vi "AddPageContent.vi"(1 "Graph last":bool=TRUE, 2 "Deckblatt":bool, 4 "TableFont":T1[](array[typedef]), 5 "HeaderTableFont":T1={"Font"="Arial", "Size"=10, "Colour"=0, "Bold"=FALSE, "Italic"=FALSE, "Underline"=FALSE, "Strikethrough"=FALSE, "Font Encoding"=enum."Cp1252, WinANSI"}, 6 "Title Font":T1={"Font"="Arial", "Size"=26, "Colour"=0, "Bold"=TRUE, "Italic"=FALSE, "Underline"=TRUE, "Strikethrough"=FALSE, "Font Encoding"=enum."Cp1252, WinANSI"}, 7 "Column Ratio left":sgl[](array[numeric]), 8 "error in":errorcluster, 9 "Graph Array":T3[](array[typedef]) {"Align (Left)" items=["Center", "Justified", "Justified All", "Left", "Right"]}, 10 "Content":T7={"Titel"="Test mit Graph PDF", "Header Table"=[["Murks:", "4711"], ["HolyShit:", "0815"]], "Table Array"=[], "Bemerkungen"=[{"Bemerkung Text"="super geiles PDF", "Align (Left)"=0, "Add Line Feeds (F:No)"=TRUE, "Font"={"Font"="Arial", "Size"=10, "Colour"=0, "Bold"=FALSE, "Italic"=FALSE, "Underline"=FALSE, "Strikethrough"=FALSE, "Font Encoding"=enum."Cp1252, WinANSI"}}, {"Bemerkung Text"="", "Align (Left)"=0, "Add Line Feeds (F:No)"=FALSE, "Font"={"Font"="Arial", "Size"=10, "Colour"=0, "Bold"=FALSE, "Italic"=FALSE, "Underline"=FALSE, "Strikethrough"=FALSE, "Font Encoding"=enum."Cp1252, WinANSI"}}, {"Bemerkung Text"="Tabelle mit optionalen Ergebnissen", "Align (Left)"=3, "Add Line Feeds (F:No)"=FALSE, "Font"={"Font"="Arial", "Size"=10, "Colour"=0, "Bold"=FALSE, "Italic"=FALSE, "Underline"=FALSE, "Strikethrough"=FALSE, "Font Encoding"=enum."Cp1252, WinANSI"}}, {"Bemerkung Text"="Graph geht ab ... ", "Align (Left)"=0, "Add Line Feeds (F:No)"=FALSE, "Font"={"Font"="Arial", "Size"=10, "Colour"=0, "Bold"=FALSE, "Italic"=FALSE, "Underline"=FALSE, "Strikethrough"=FALSE, "Font Encoding"=enum."Cp1252, WinANSI"}}]} {"Table Array"."Horizontal Align" items=["Center", "Justified", "JustifiedAll", "Left", "Right"]; "Table Array"."TablePictures"."Horizontal Align" items=["Center", "Justified", "JustifiedAll", "Left", "Right"]; "Table Array"."Results"."Position" items=["First", "Last"]; "Table Array"."Results"."Horizontal Align" items=["Center", "Justified", "JustifiedAll", "Left", "Right"]; "Bemerkungen"."Align (Left)" items=["Center", "Justified", "Justified All", "Left", "Right"]}, 11 "Context (Eingang)":refnum<class "Context.lvclass">) -> (0 "error out":errorcluster, 3 "Context (Ausgang)":refnum<class "Context.lvclass">)   [LabVIEW 2020, in "PDF Interface.lvlib"]
doc: "To add Content to a PDF Page that was created by \"InitBeforePage\" or after \"AddAdditionalPage\"."
uses:
  PDF Interface.lvlib
  <vilib>/Simplicity AI/SAI_PDF_API/Classes/Context/Controls/SAI_PDF_Font.ctl
  <vilib>/Simplicity AI/SAI_PDF_API/Classes/Context/Controls/SAI_PDF_Font Encoding.ctl
  PDF Interface Helper/PDFContentType.ctl
  PDF Interface Helper/PDFTableContentType.ctl
  PDF Interface Helper/PDFResults.ctl
  PDF Interface Helper/PDFResultPictures.ctl
  PDF Interface Helper/PDFCommentPosition.ctl
  PDF Interface Helper/PDFPageBreak.ctl
  PDF Interface Helper/PDFTablePictures.ctl
  PDF Interface Helper/PDFBemerkung.ctl
  <vilib>/Simplicity AI/SAI_PDF_API/Classes/Context/Controls/SAI_PDF_Text Align.ctl
  PDF Interface Helper/PDFGraph.ctl
  <vilib>/Simplicity AI/SAI_PDF_API/Classes/Context/Context.lvclass
  PDF Interface Helper/PDF Interface Helper.lvlib
panel:
  # "(Cp1252)"
  # "(Cp1252)"
  # "(Cp1252)"
  # "(Cp1252)"
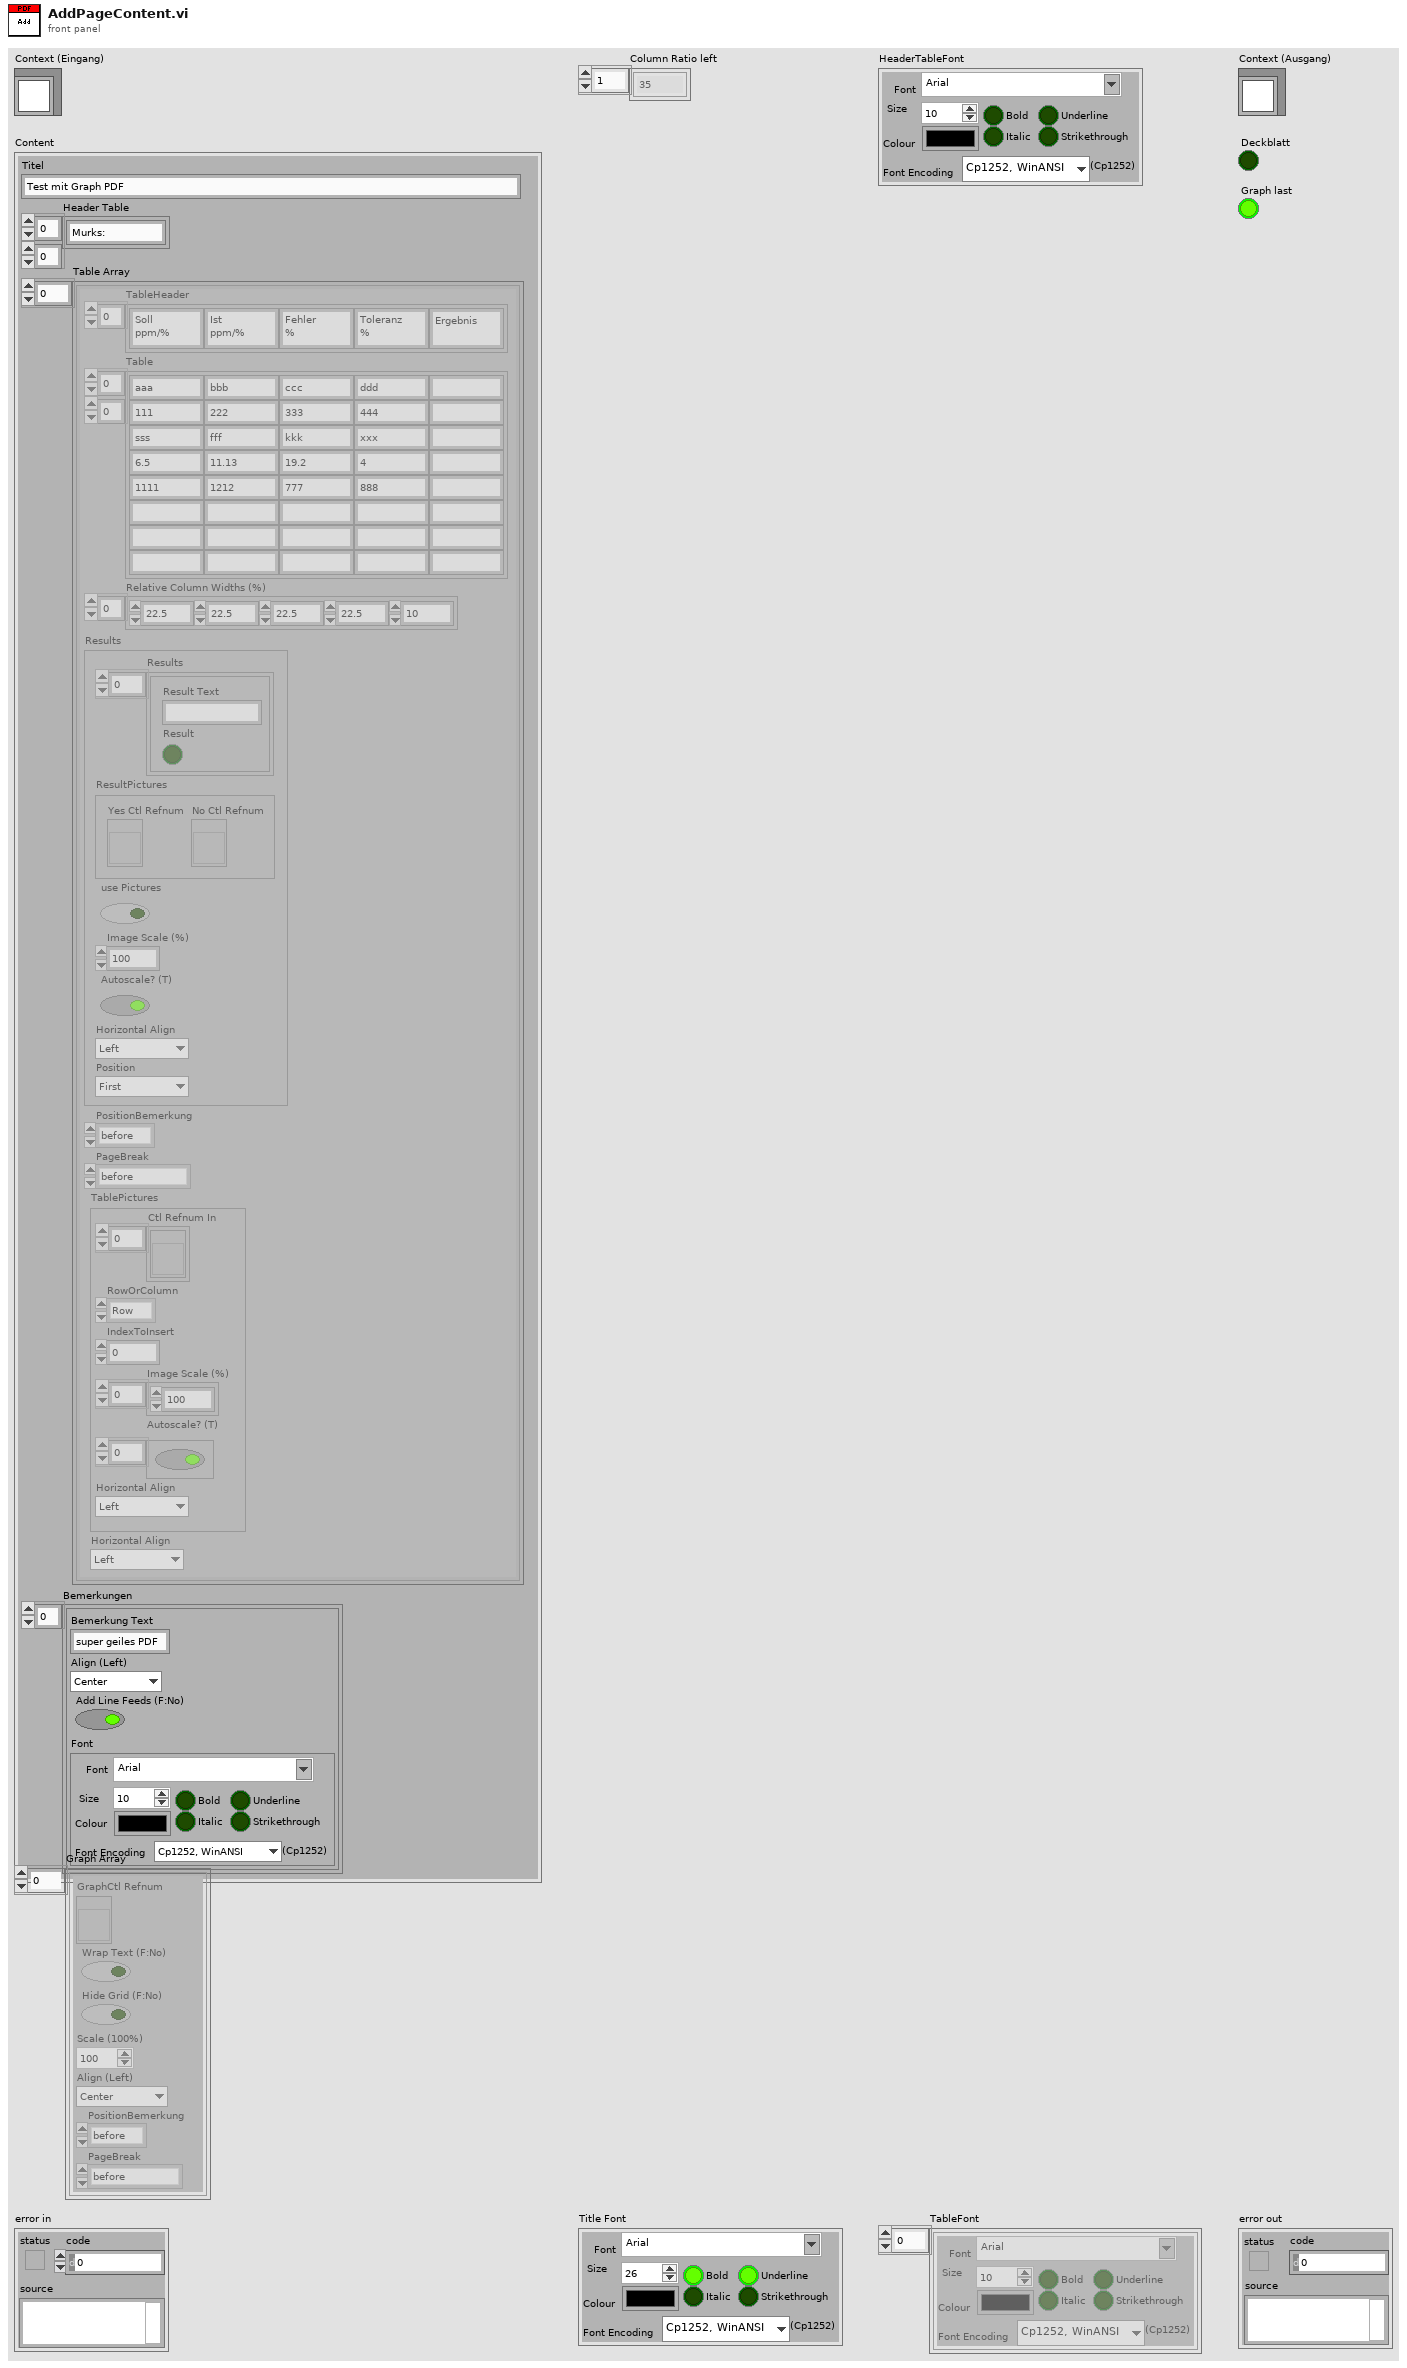
[diagram p1: front panel]
types:
  T1 = typedef "SAI_PDF_Toolkit.lvlib/Context.lvclass/SAI_PDF_Font.ctl" = cluster{"Font":string, "Size":i32, "Colour":u32, "Bold":bool, "Italic":bool, "Underline":bool, "Strikethrough":bool, "Font Encoding":T2}
  T2 = typedef "SAI_PDF_Toolkit.lvlib/Context.lvclass/SAI_PDF_Font Encoding.ctl" = enum16{"Cp1252, WinANSI", "IdentityH", "IdentityV", "Cp1250", "Cp1257", "MacRoman"}
  T3 = typedef "PDF Interface.lvlib/PDF Interface Helper.lvlib/PDFGraph.ctl" = cluster{"GraphCtl Refnum":refnum<vi>, "Wrap Text (F:No)":bool, "Hide Grid (F:No)":bool, "Scale (100%)":sgl, "Align (Left)":T4, "PositionBemerkung":T5, "PageBreak":T6}
  T4 = typedef "SAI_PDF_Toolkit.lvlib/Context.lvclass/SAI_PDF_Text Align.ctl" = i32
  T5 = typedef "PDF Interface.lvlib/PDF Interface Helper.lvlib/PDFCommentPosition.ctl" = enum16{"before", "after"}
  T6 = typedef "PDF Interface.lvlib/PDF Interface Helper.lvlib/PDFPageBreak.ctl" = enum16{"none", "before", "after", "after comment"}
  T7 = typedef "PDF Interface.lvlib/PDF Interface Helper.lvlib/PDFContentType.ctl" = cluster{"Titel":string, "Header Table":string[][], "Table Array":T8[], "Bemerkungen":T12[]}
  T8 = typedef "PDF Interface.lvlib/PDF Interface Helper.lvlib/PDFTableContentType.ctl" = cluster{"TableHeader":string[], "Table":string[][], "Relative Column Widths (%)":sgl[], "Results":T9, "PositionBemerkung":T5, "PageBreak":T6, "TablePictures":T11, "Horizontal Align":i32}
  T9 = typedef "PDF Interface.lvlib/PDF Interface Helper.lvlib/PDFResults.ctl" = cluster{"Results":cluster{"Result Text":string, "Result":bool}[], "ResultPictures":T10, "use Pictures":bool, "Image Scale (%)":sgl, "Autoscale? (T)":bool, "Horizontal Align":i32, "Position":i32}
  T10 = typedef "PDF Interface.lvlib/PDF Interface Helper.lvlib/PDFResultPictures.ctl" = cluster{"Yes Ctl Refnum":refnum<vi>, "No Ctl Refnum":refnum<vi>}
  T11 = typedef "PDF Interface.lvlib/PDF Interface Helper.lvlib/PDFTablePictures.ctl" = cluster{"Ctl Refnum In":refnum<vi>[], "RowOrColumn":enum16{"Row", "Column"}, "IndexToInsert":u16, "Image Scale (%)":sgl[], "Autoscale? (T)":bool[], "Horizontal Align":i32}
  T12 = typedef "PDF Interface.lvlib/PDF Interface Helper.lvlib/PDFBemerkung.ctl" = cluster{"Bemerkung Text":string, "Align (Left)":T4, "Add Line Feeds (F:No)":bool, "Font":T1}
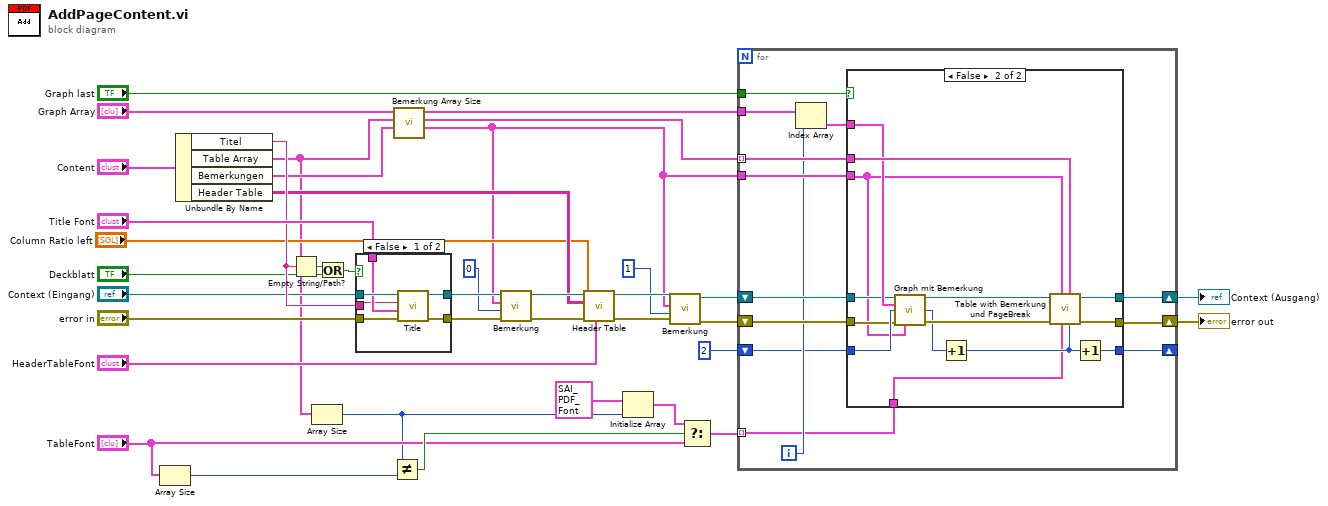
[diagram p0: block diagram]
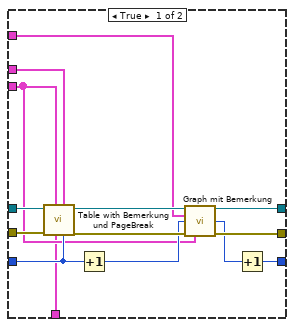
[diagram p2: hidden frame]
diagram:
  n1 = Array Size(array="TableFont") -> (size(s)=w6:i32)
  n2 = Unbundle By Name("Content") -> ("Titel"=w23:string, "Table Array"=w8:T8[], "Bemerkungen"=w12:T12[], "Header Table"=w21:string[][])
  n3 = Empty String/Path?(string/path=w23) -> (empty?=w22:bool)
  n4 = Array Size(array=w8) -> (size(s)=w1:i32)
  n5 = Or(x=w22, y="Deckblatt") -> (x .or. y?=w16:bool)
  n6 = case shown="False" w16 {
    tunnel: [w44 w46] -> w38
    tunnel: [w43 w45] -> w37
    tunnel: "error in" -> [w42 w45]
    tunnel: "Context (Eingang)" -> [w41 w46]
    tunnel: "Title Font" -> [w40 _]
    tunnel: w23 -> [w39 _]
    frame False {
      n7 = call "Title.vi"("error in (no error)"=w42, "Font"=w40, "Text"=w39, "Context in"=w41) -> ("error out"=w43:errorcluster, "Context out"=w44:refnum<class "Context.lvclass">)  [unwired: 3 in, 3 out]
    }
    frame True {
    }
  }
  n8 = Not Equal?(x=w1, y=w6) -> (x != y?=w5:bool)
  n9 = call "Bemerkung Array Size.vi"("Bemerkungen (Eingang)"=w12, "Table Array (Eingang)"=w8, "Graph Array (Eingang)"="Graph Array") -> ("Bemerkungen (Ausgang)"=w9:T12[], "Table Array (Ausgang)"=w10:T8[], "Graph Array (Ausgang)"=w11:T3[])  [unwired: 5 in, 1 out]
  n10 = call "Bemerkung.vi"("Fehler (Eingang, kein Fehler)"=w37, "Index"=0, "Bemerkung"=w9, "Context (Eingang)"=w38) -> ("Fehler (Ausgang)"=w35:errorcluster, "Context (Ausgang)"=w36:refnum<class "Context.lvclass">)  [unwired: 6 in]
  n11 = call "Header Table.vi"("Font"="HeaderTableFont", "error in"=w35, "Column Ratio left"="Column Ratio left", "Table"=w21, "Context In"=w36) -> ("error out"=w26:errorcluster, "Context Out"=w29:refnum<class "Context.lvclass">)  [unwired: 5 in]
  n12 = Initialize Array(T1 {"Font"="Arial", "Size"=10, "Colour"=0, "Bold"=FALSE, "Italic"=FALSE, "Underline"=FALSE, "Strikethrough"=FALSE, "Font Encoding"=enum."Cp1252, WinANSI"} ("TableFont"), w1) -> (w4:T1[])
  n13 = call "Bemerkung.vi"("Fehler (Eingang, kein Fehler)"=w26, "Index"=1, "Bemerkung"=w9, "Context (Eingang)"=w29) -> ("Fehler (Ausgang)"=w27:errorcluster, "Context (Ausgang)"=w28:refnum<class "Context.lvclass">)  [unwired: 6 in]
  n14 = Select(t=w4, s=w5, f="TableFont") -> (s? t:f=w2:T1[])
  n15 = for {
    tunnel: w11 -> [w53]
    tunnel: w9 -> [w55]
    tunnel: w10 -> [w54] mode=indexing
    shift-right: [w59] -> w31
    shift-left: w28 -> [w57]
    shift-right: [w58] -> w30
    shift-left: w27 -> [w56]
    shift-right: [w50] -> _
    shift-left: 2 ("Index") -> [w51]
    tunnel: "Graph last" -> [w48]
    tunnel: w2 -> [w47] mode=indexing
    i -> [w52]
    n16 = Index Array(array=w53, index=w52) -> (element=w49:T3)
    n17 = case shown="False" w48 {
      tunnel: [w72 w77] -> w59
      tunnel: [w70 w76] -> w58
      tunnel: w57 -> [w69 w83]
      tunnel: w56 -> [w68 w82]
      tunnel: w55 -> [w61 w75]
      tunnel: w54 -> [w67 w87]
      tunnel: w51 -> [w66 w84]
      tunnel: [w65 w86] -> w50
      tunnel: w49 -> [w63 w85]
      tunnel: w47 -> [w60 w74]
      frame True {
        n18 = call "Table with Bemerkung und PageBreak.vi"("Index"=w66, "Table Content"=w67, "TableFont"=w60, "Bemerkungen"=w61, "Fehler (Eingang, kein Fehler)"=w68, "Context (Eingang)"=w69) -> ("Fehler (Ausgang)"=w71:errorcluster, "Context (Ausgang)"=w73:refnum<class "Context.lvclass">)  [unwired: 4 in]
        n19 = Increment(x=w66) -> (x+1=w64:i32)
        n20 = call "Graph mit Bemerkung.vi"("Context (Eingang)"=w73, "Graph"=w63, "Bemerkung Index (Eingang)"=w64, "Fehler (Eingang, kein Fehler)"=w71, "Bemerkungen"=w61) -> ("Context (Ausgang)"=w72:refnum<class "Context.lvclass">, "Bemerkung Index (Ausgang)"=w62:i32, "Fehler (Ausgang)"=w70:errorcluster)  [unwired: 8 in]
        n21 = Increment(x=w62) -> (x+1=w65:i32)
      }
      frame False {
        n22 = call "Graph mit Bemerkung.vi"("Context (Eingang)"=w83, "Graph"=w85, "Bemerkung Index (Eingang)"=w84, "Fehler (Eingang, kein Fehler)"=w82, "Bemerkungen"=w75) -> ("Context (Ausgang)"=w81:refnum<class "Context.lvclass">, "Bemerkung Index (Ausgang)"=w79:i32, "Fehler (Ausgang)"=w80:errorcluster)  [unwired: 8 in]
        n23 = Increment(x=w79) -> (x+1=w78:i32)
        n24 = call "Table with Bemerkung und PageBreak.vi"("Index"=w78, "Table Content"=w87, "TableFont"=w74, "Bemerkungen"=w75, "Fehler (Eingang, kein Fehler)"=w80, "Context (Eingang)"=w81) -> ("Fehler (Ausgang)"=w76:errorcluster, "Context (Ausgang)"=w77:refnum<class "Context.lvclass">)  [unwired: 4 in]
        n25 = Increment(x=w78) -> (x+1=w86:i32)
      }
    }
  }
  "error out" <- w30
  "Context (Ausgang)" <- w31
